vi "Personnel API Test.vi"() -> ()   [LabVIEW 2015]
uses:
  LVRestAPI/TypeDef/FGVAction.ctl
  LVRestAPI/RoomRestApi.lvlib
  LVRestAPI/PersonnelRestApi.lvlib
panel:
  in  "PUID":string
  out "Response":string
  out "Error Out":errorcluster
  in  "Refresh Button":bool
  in  "Room":i32
  in  "Out of Room":bool
  in  "Into Room":bool
  in  "stop":bool
  in  "URL":string="http://127.0.0.1:8001/RivERWebService/"
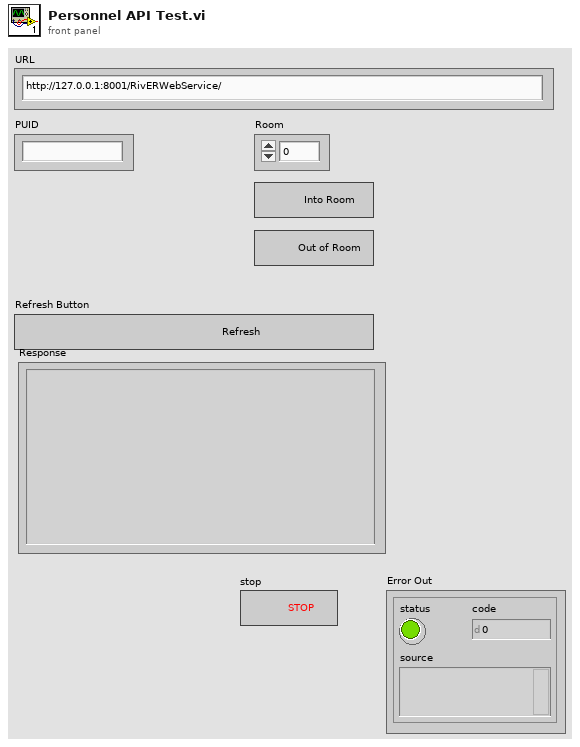
[diagram p1: front panel]
types:
  T1 = typedef "RoomRestApi.lvlib/FGVAction.ctl" = enum16{"Get", "Set"}
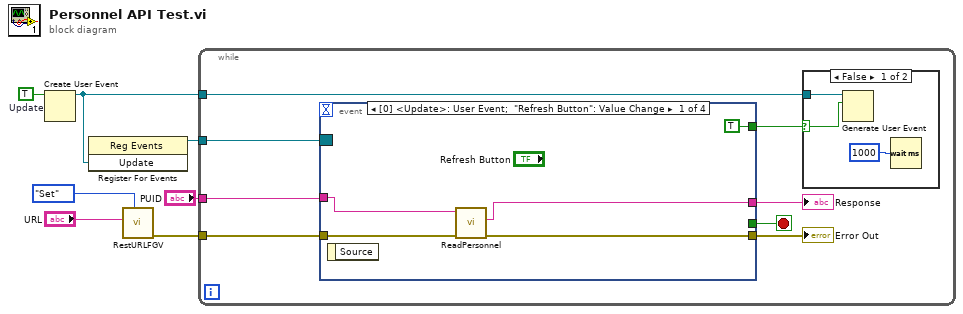
[diagram p0: block diagram]
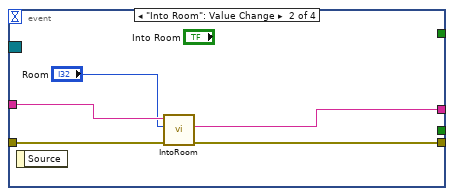
[diagram p3: hidden frame]
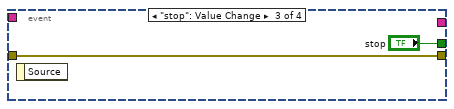
[diagram p4: hidden frame]
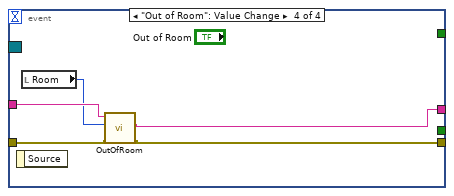
[diagram p5: hidden frame]
diagram:
  w4 = TRUE  # Update
  n1 = Create User Event(user event datatype=w4) -> (user event=w3:refnum<user-event>)  [unwired: 1 in, 1 out]
  n2 = register-events(w3) -> (reference out=w2:refnum<event-registration>)  [unwired: 2 in, 1 out]
  n3 = call "RestURLFGV.vi"("Action"=FGVAction."Set", "URL"="URL") -> ("error out"=w5:errorcluster)  [unwired: 8 in, 1 out]
  n4 = while {
    tunnel: w5 -> [w15]
    tunnel: w3 -> [w10]
    tunnel: w2 -> [w9]
    tunnel: "PUID" -> [w8]
    stop <- w12 stop-if-true
    n5 = event shown="[0] <Update>: User Event;  \"Refresh Button\": Value Change" {
      selector: w9 -> [_ _ _ _]
      dyn-events: _ -> [_ _ _ _]
      timeout: _ -> [_ _ _ _]
      tunnel: w15 -> [w22 w27 w29 w34]
      tunnel: [w21 w26 w29 w33] -> w14
      tunnel: [w19 w25 _ w32] -> w13
      tunnel: w8 -> [w20 w28 _ w35]
      tunnel: [_ _ "stop" _] -> w12
      tunnel: [TRUE _ _ _] -> w11
      event User Event; "Refresh Button": Value Change {
        n6 = event-data() -> ()  [unwired: 1 in, 1 out]
        n7 = call "ReadPersonnel.vi"("error in (no error)"=w22, "PUID"=w20) -> ("error out"=w21:errorcluster, "Personnel"=w19:string)  [unwired: 8 in]
      }
      event "Into Room": Value Change {
        n8 = event-data() -> ()  [unwired: 1 in, 1 out]
        n9 = call "IntoRoom.vi"("error in (no error)"=w27, "Room"="Room", "PUID"=w28) -> ("error out"=w26:errorcluster, "Response"=w25:string)  [unwired: 7 in]
      }
      event "stop": Value Change {
        n10 = event-data() -> ()  [unwired: 1 in, 1 out]
      }
      event "Out of Room": Value Change {
        n11 = event-data() -> ()  [unwired: 1 in, 1 out]
        n12 = local read "Room"() -> (w31:i32)
        n13 = call "OutOfRoom.vi"("error in (no error)"=w34, "Room"=w31, "PUID"=w35) -> ("error out"=w33:errorcluster, "Response"=w32:string)  [unwired: 7 in]
      }
    }
    "Response" <- w13
    "Error Out" <- w14
    n14 = case shown="False" w11 {
      selector: w11 -> [w16 _]
      tunnel: w10 -> [w17 _]
      frame False {
        n15 = Generate User Event(user event=w17, event data cluster=w16) -> ()  [unwired: 2 in, 2 out]
        n16 = Wait (ms)(milliseconds to wait=u32 1000) -> ()  [unwired: 1 out]
      }
      frame True {
      }
    }
  }
